vi "Remove Single Node.vi"(8 "error in (no error)":errorcluster, 9 "Actor ID":variant, 10 "Timeout(ms)":i64=3000, 11 "Simple Numeric Map Node Controller in":refnum<class "Simple Numeric Map Node Controller.lvclass">) -> (0 "error out":errorcluster, 3 "Simple Numeric Map Node Controller out":refnum<class "Simple Numeric Map Node Controller.lvclass">)   [LabVIEW 2024, in "Simple Numeric Map Node Controller.lvclass"]
uses:
  Simple Numeric Map Node Controller.lvclass
  Simple Numeric Map Node Controller.lvclass/Simple Numeric Map Node Controller.ctl
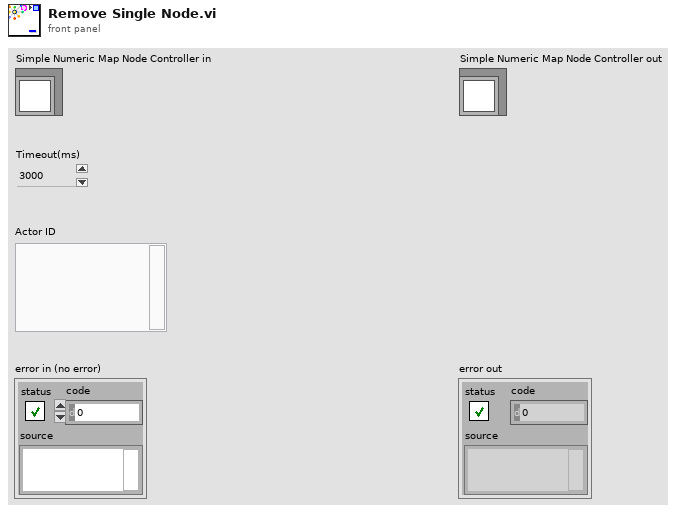
[diagram p1: front panel]
types:
  T1 = enum32{"Bad", "Idle", "Run top level", "Running"}
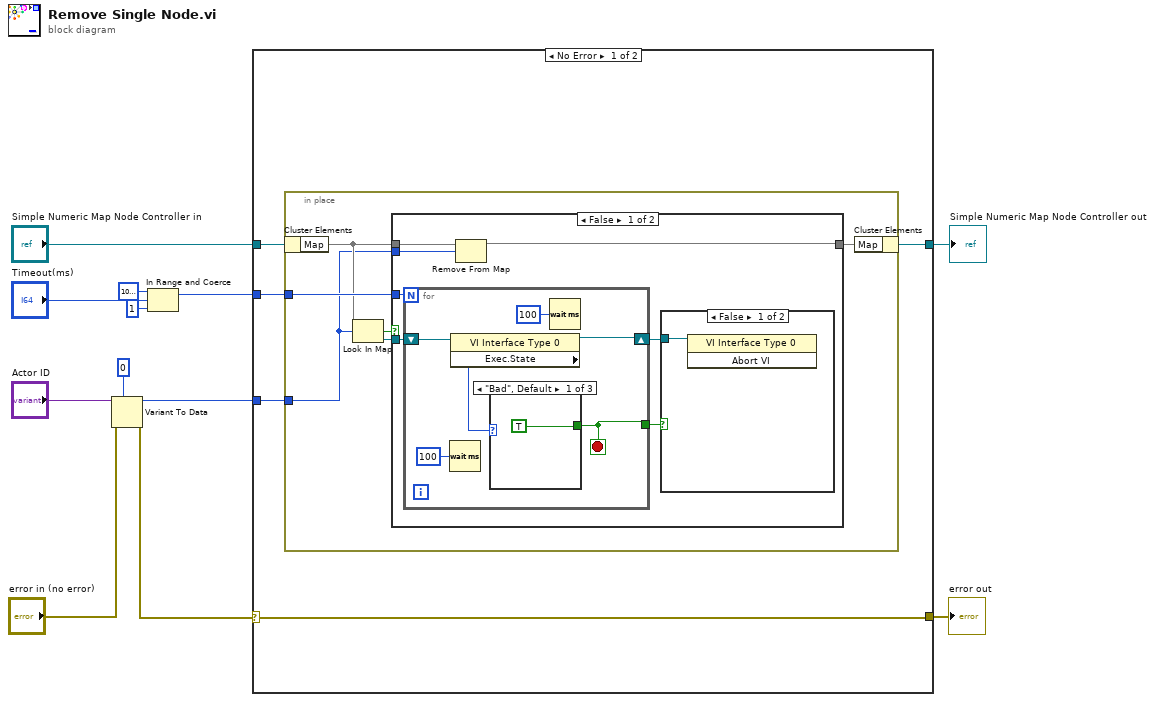
[diagram p0: block diagram]
diagram:
  n1 = Variant To Data(error in="error in (no error)", type=i64 0 ("Timeout(ms)"), Variant="Actor ID") -> (data=w5:i64, error out=w9:errorcluster)
  n2 = In Range and Coerce(upper limit=i64 1000000000, x="Timeout(ms)", lower limit=i64 1) -> (coerced(x)=w1:i64)  [unwired: 1 out]
  n3 = case shown="No Error" w9 {
    selector: w9 -> [w17 w40]
    tunnel: "Simple Numeric Map Node Controller in" -> [w16 w41]
    tunnel: [w15 w41] -> w7
    tunnel: [w17 w40] -> w6
    tunnel: w5 -> [w14 _]
    tunnel: w1 -> [w13 _]
    frame No Error {
      n4 = in-place {
        in-place-border: w14 -> [w18]
        in-place-border: w13 -> [w21]
        n5 = in-place-cluster #1(w16) -> ("Map"=w19:map{i64, refnum<vi>})
        n6 = Look In Map(map=w19, key=w18) -> (key not found?=w22:bool, value=w23:refnum<vi>)  [unwired: 1 in]
        n7 = case shown="False" w22 {
          tunnel: w23 -> [w30 _]
          tunnel: w21 -> [w27 _]
          tunnel: [w25 w39] -> w20
          tunnel: w19 -> [w26 w39]
          tunnel: w18 -> [w24 _]
          frame False {
            n8 = for {
              N: w27 -> [_]
              shift-right: [w35] -> w29
              shift-left: w30 -> [w36]
              tunnel: [w33] -> w28
              stop <- w33 stop-if-true
              n9 = Wait (ms)(milliseconds to wait=u32 100) -> ()  [unwired: 1 out]
              n10 = property class="VI Interface Type 0"(reference=w36) -> (reference out=w35:refnum<vi>, "Exec.State"=w34:T1)  [unwired: 1 in, 1 out]
              n11 = case shown="\"Bad\", Default" w34 {
                tunnel: [TRUE _ _] -> w33
                frame "Bad", Default {
                }
                frame "Run top level" {
                }
                frame "Running" {
                }
              }
              n12 = Wait (ms)(milliseconds to wait=u32 100) -> ()  [unwired: 1 out]
            }
            n13 = Remove From Map(10:w24, 11:w26) -> (3:w25:map{i64, refnum<vi>})  [unwired: 2 out]
            n14 = case shown="False" w28 {
              tunnel: w29 -> [w31 _]
              frame False {
                n15 = invoke class="VI Interface Type 0" method="Abort VI"(reference=w31) -> ()  [unwired: 2 in, 3 out]
              }
              frame True {
              }
            }
          }
          frame True {
          }
        }
        n16 = in-place-cluster #1("Map"=w20) -> (w15:refnum<class "Simple Numeric Map Node Controller.lvclass">)
      }
    }
    frame Error {
    }
  }
  "error out" <- w6
  "Simple Numeric Map Node Controller out" <- w7
